vi "Initialize Communication References.vi"() -> (0 "error out":errorcluster, 2 "Processing Loop Queue":refnum<queue>, 3 "Event Registration Refnum":refnum<event-registration>)   [LabVIEW 2013, in "LVTM.lvlib"]
uses:
  LVTM.lvlib
  Controls_LVTM/RequestEvents.ctl
  Controls_LVTM/UserEventDataPause.ctl
  Controls_LVTM/UserEventUpdateTreeItems.ctl
panel:
  in  "error in":errorcluster
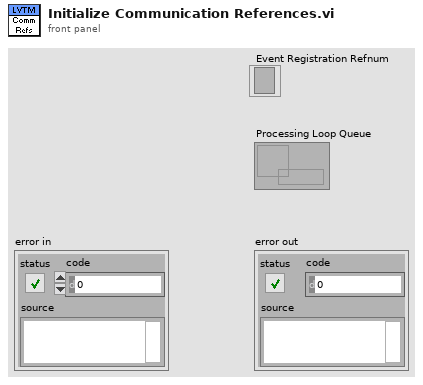
[diagram p1: front panel]
types:
  T1 = typedef "LVTM.lvlib/RequestEvents.ctl" = cluster{"Pause":refnum<user-event>, "Handle Error":refnum<user-event>, "Update Items":refnum<user-event>}
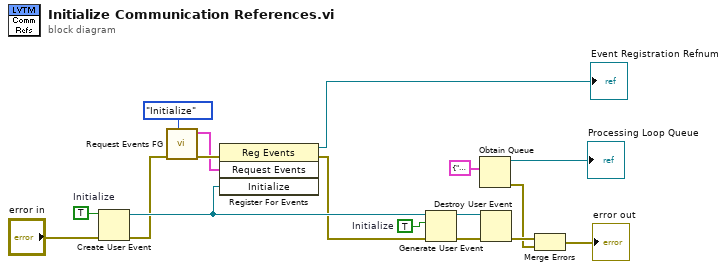
[diagram p0: block diagram]
diagram:
  w14 = TRUE  # Initialize
  w13 = TRUE  # Initialize
  n1 = Create User Event(user event datatype=w13, error in="error in") -> (user event=w17:refnum<user-event>, error out=w15:errorcluster)
  n2 = call "Request Events FG.vi"("Action (Get)"=enum16{"Initialize", "Get", "Destroy"}."Initialize" ("Action"), "error in"=w15) -> ("error out"=w12:errorcluster, "Request Events"=w10:T1)  [unwired: 8 in]
  n3 = register-events(error in=w12, w10, w17) -> (reference out=→"Event Registration Refnum":refnum<event-registration>, error out=w16:errorcluster)  [unwired: 1 in]
  n4 = Generate User Event(user event=w17, event data cluster=w14, error in=w16) -> (user event out=w7:refnum<user-event>, error out=w6:errorcluster)  [unwired: 1 in]
  n5 = Obtain Queue(element data type=cluster{"Command":string, "Data":variant} {"Command"="", "Data"=variant}) -> (queue out=→"Processing Loop Queue":refnum<queue>, error out=w1:errorcluster)  [unwired: 4 in, 1 out]
  n6 = Destroy User Event(user event=w7, error in=w6) -> (error out=w5:errorcluster)
  n7 = Merge Errors(w5, w1) -> (→"error out":errorcluster)
